vi "CalculateTrajectory2.vi"(9 "ChangingDistance":dbl, 10 "Inputs":T1, 11 "Lanes":T2) -> (2 "Trajectory":cluster{"X":dbl[], "Y":dbl[], "Theta":dbl[]})   [LabVIEW 2013]
uses:
  <vilib>/imath/engines/lvmath2/RunTimeEngine/ErrorHandling/NIMS_Finalize Error.vi
  <vilib>/imath/engines/lvmath2/RunTimeEngine/Managers/WorkSpace/UID Generator.vi
  <vilib>/imath/engines/lvmath2/RunTimeEngine/IndexRead/NIMS M($,S).vi
  <instcachedir>/0/NIMS M($,S)_3E5749BBB62E49528D4765A77F1F6D98.lvgen/NIMS M($,S)_3E5749BBB62E49528D4765A77F1F6D98_000.vi
  <vilib>/imathl/engines/lvmath/Functions/Error Handling/Create Error.vi
  <vilib>/imath/engines/lvmath2/RunTimeEngine/CommandStatement/NIMS_CommandStatement_MaskErr.vi
  <vilib>/imath/engines/lvmath2/RunTimeEngine/Managers/SymbolTable/Clear UID.vi
  <vilib>/imath/engines/lvmath2/RunTimeEngine/NodeEndStatement/NIMS_NodeEndStatement_Output.vi
  <instcachedir>/0/NIMS_NodeEndStatement_Output_53EC0D466D134D7ABD903AC30B43404B.lvgen/NIMS_NodeEndStatement_Output_53EC0D466D134D7ABD903AC30B43404B_005.vi
  <instcachedir>/0/NIMS_NodeEndStatement_Output_53EC0D466D134D7ABD903AC30B43404B.lvgen/NIMS_NodeEndStatement_Output_53EC0D466D134D7ABD903AC30B43404B_000.vi
  <vilib>/imath/engines/lvmath2/RunTimeEngine/IndexRead/NIMS V(S).vi
  <instcachedir>/0/NIMS V(S)_0488751826AF41519A22953C041130DC.lvgen/NIMS V(S)_0488751826AF41519A22953C041130DC_000.vi
  <vilib>/imath/engines/lvmath2/RunTimeEngine/ArithmeticOperatorToken/NIMS_ArithmeticOperator_plus.vi
  <instcachedir>/0/NIMS_ArithmeticOperator_plus_8A46DAFC24D445C9B2C97B626139369E.lvgen/NIMS_ArithmeticOperator_plus_8A46DAFC24D445C9B2C97B626139369E_004.vi
  <vilib>/imath/engines/lvmath2/RunTimeEngine/ErrorHandling/NIMS_Create Error From Enums.vi
  <vilib>/imath/engines/lvmath2/RunTimeEngine/BuiltInFunctions/min/1 input/NIMS_min(CV).vi
  <instcachedir>/0/NIMS_min(CV)_46E60952406B4159AB512BDF500C959F.lvgen/NIMS_min(CV)_46E60952406B4159AB512BDF500C959F_000.vi
  <vilib>/imath/engines/lvmath2/RunTimeEngine/CommandStatement/MC_CommandStatement_break.vi
  <vilib>/imath/engines/lvmath2/RunTimeEngine/BuiltInFunctions/length/NIMS_length(GV).vi
  <instcachedir>/0/NIMS_length(GV)_08A3D13377FD4E4B96F5795FBF3698FA.lvgen/NIMS_length(GV)_08A3D13377FD4E4B96F5795FBF3698FA_000.vi
  <vilib>/imath/engines/lvmath2/RunTimeEngine/IndexRead/NIMS V(R2).vi
  <instcachedir>/0/NIMS V(R2)_C76619605A0E4E9F8B2FA9389712AC47.lvgen/NIMS V(R2)_C76619605A0E4E9F8B2FA9389712AC47_000.vi
  <vilib>/imath/engines/lvmath2/RunTimeEngine/RunTimeType/NIMS_RunTimeType_From StrictType (excl LVString).vi
  <instcachedir>/0/NIMS_RunTimeType_From StrictType (excl LVString)_4DEE718D6EB74582AA20236969C084FC.lvgen/NIMS_RunTimeType_From StrictType (excl LVString)_4DEE718D6EB74582AA20236969C084FC_000.vi
  <vilib>/imath/engines/lvmath2/RunTimeEngine/LocalVariableDefStatement/MC_LocalVariableDefStatement_Display.vi
  <vilib>/imath/engines/lvmath2/RunTimeEngine/RangeToken/NIMS_Range.vi
  <instcachedir>/0/NIMS_Range_7481B155BEE341ECA0F59DDB444E2C09.lvgen/NIMS_Range_7481B155BEE341ECA0F59DDB444E2C09_000.vi
  <vilib>/imath/engines/lvmath2/RunTimeEngine/ArithmeticOperatorToken/NIMS_ArithmeticOperator_times.vi
  <instcachedir>/0/NIMS_ArithmeticOperator_times_F6527734CE75451889337B8CE94765C6.lvgen/NIMS_ArithmeticOperator_times_F6527734CE75451889337B8CE94765C6_002.vi
  <instcachedir>/0/NIMS_ArithmeticOperator_plus_8A46DAFC24D445C9B2C97B626139369E.lvgen/NIMS_ArithmeticOperator_plus_8A46DAFC24D445C9B2C97B626139369E_001.vi
  <vilib>/imath/engines/lvmath2/RunTimeEngine/BuiltInFunctions/difference/NIMS_difference(GV,I32).vi
  <instcachedir>/0/NIMS_difference(GV,I32)_DC7351DCBCF840A8AE147F50EC2CE86E.lvgen/NIMS_difference(GV,I32)_DC7351DCBCF840A8AE147F50EC2CE86E_001.vi
  <vilib>/imath/engines/lvmath2/RunTimeEngine/BuiltInFunctions/atan2/NIMS_atan2(A,A).vi
  <instcachedir>/0/NIMS_atan2(A,A)_2936FD7F864E46C682B467FE18724EF9.lvgen/NIMS_atan2(A,A)_2936FD7F864E46C682B467FE18724EF9_005.vi
  <vilib>/imath/engines/lvmath2/RunTimeEngine/Managers/SymbolTable/NIMS_WorkSpace.lvlib
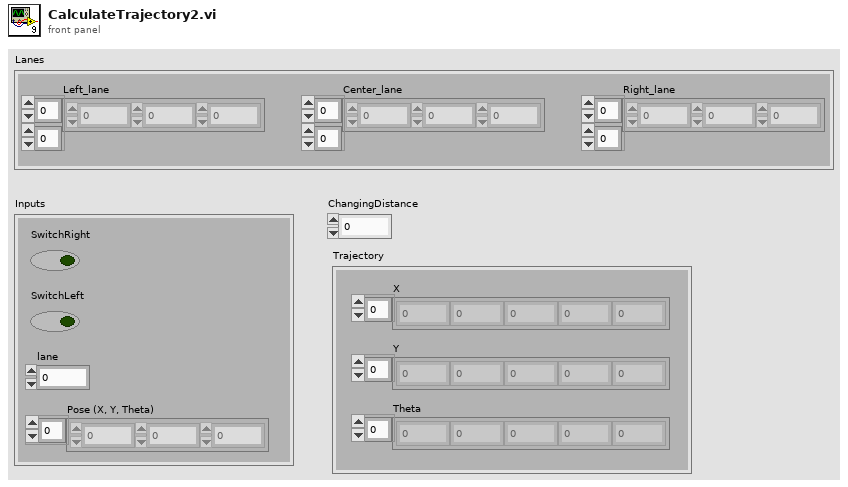
[diagram p1: front panel]
types:
  T1 = cluster{"Pose (X, Y, Theta)":dbl[], "lane":dbl, "SwitchRight":bool, "SwitchLeft":bool}
  T2 = cluster{"Right_lane":dbl[][], "Center_lane":dbl[][], "Left_lane":dbl[][]}
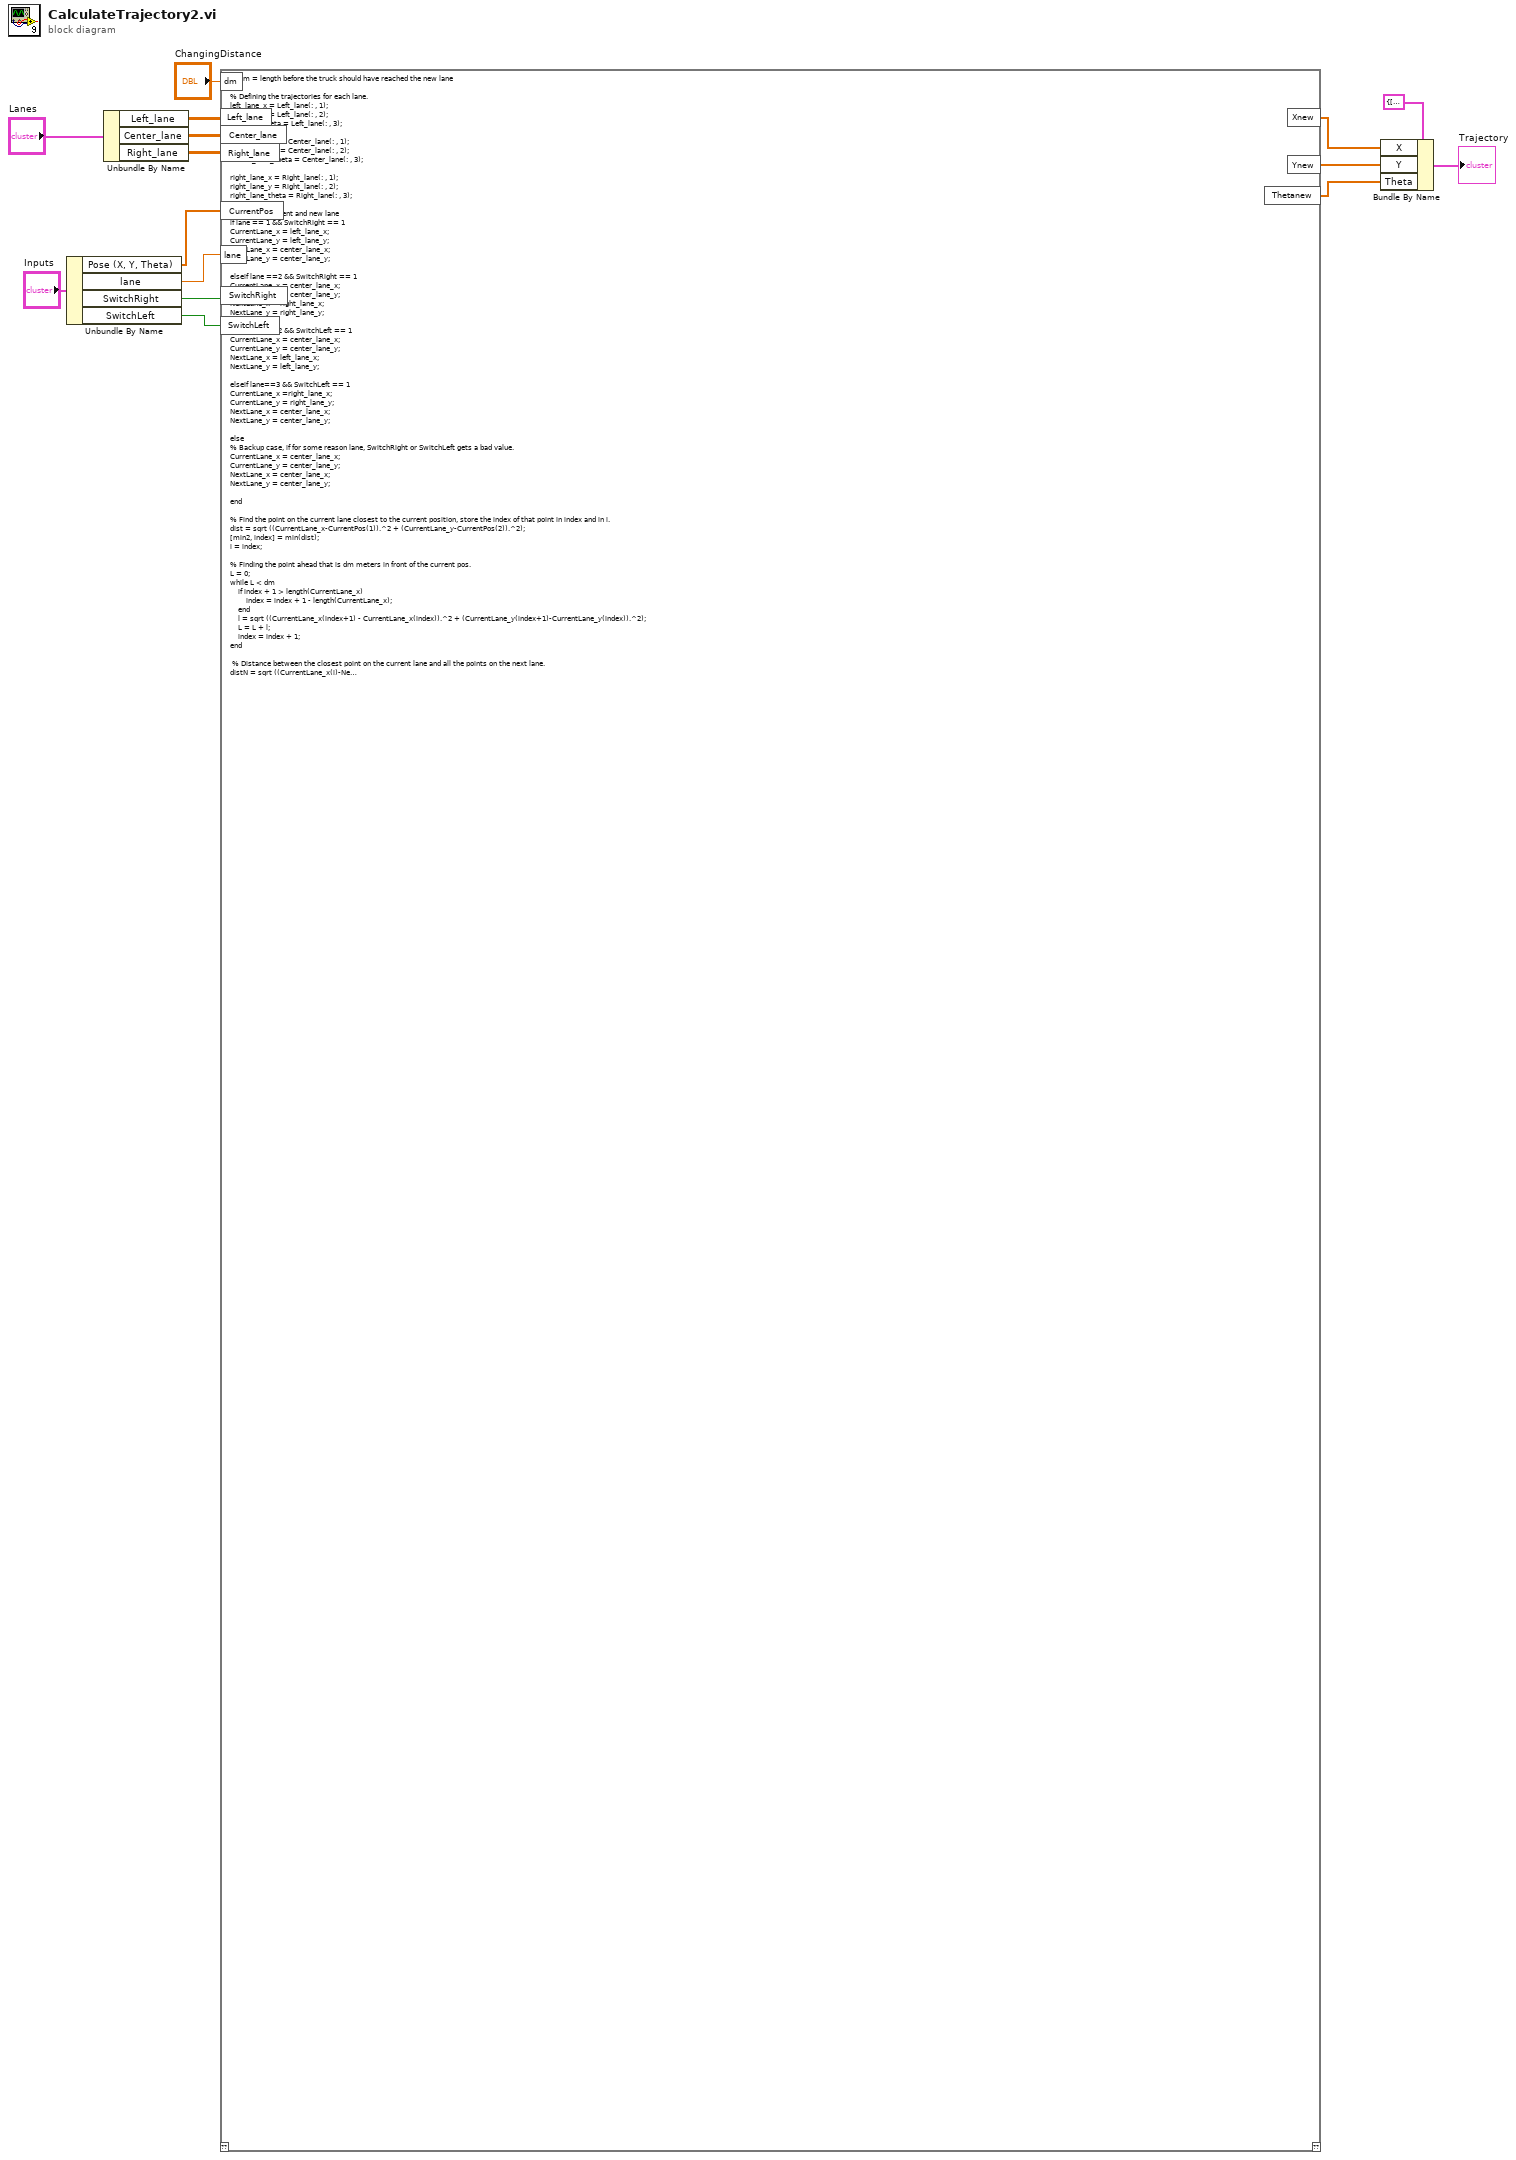
[diagram p0: block diagram]
diagram:
  n1 = Unbundle By Name("Inputs") -> ("Pose (X, Y, Theta)"=w11:dbl[], "lane"=w10:dbl, "SwitchRight"=w9:bool, "SwitchLeft"=w8:bool)
  n2 = Unbundle By Name("Lanes") -> ("Left_lane"=w15:dbl[][], "Center_lane"=w14:dbl[][], "Right_lane"=w13:dbl[][])
  n3 = mathscript code="% dm = length before the truck should have reached the new lane\n\n% Defining the trajectories for each lane.\nleft_lane_x = Left_lane(: , 1);\nleft_lane_y = Left_lane(: , 2);\nleft_lane_theta = Left_lane(: , 3);\n\ncenter_lane_x = Center_lane(: , 1);\ncenter_lane_y = Center_lane(: , 2);\ncenter_lane_theta = Center_lane(: , 3);\n\nright_lane_x = Right_lane(: , 1);\nright_lane_y = Right_lane(: , 2);\nright_lane_theta = Right_lane(: , 3);\n\n% Defining current and new lane\nif lane == 1 && SwitchRight == 1\nCurrentLane_x = left_lane_x;\nCurrentLane_y = left_lane_y;\nNextLane_x = center_lane_x;\nNextLane_y = center_lane_y;\n\nelseif lane ==2 && SwitchRight == 1\nCurrentLane_x = center_lane_x;\nCurrentLane_y = center_lane_y;\nNextLane_x = right_lane_x;\nNextLane_y = right_lane_y;\n\nelseif lane ==2 && SwitchLeft == 1\nCurrentLane_x = center_lane_x;\nCurrentLane_y = center_lane_y;\nNextLane_x = left_lane_x;\nNextLane_y = left_lane_y;\n\nelseif lane==3 && SwitchLeft == 1\nCurrentLane_x =right_lane_x;\nCurrentLane_y = right_lane_y;\nNextLane_x = center_lane_x;\nNextLane_y = center_lane_y;\n\nelse\n% Backup case, if for some reason lane, SwitchRight or SwitchLeft gets a bad value. \nCurrentLane_x = center_lane_x;\nCurrentLane_y = center_lane_y;\nNextLane_x = center_lane_x;\nNextLane_y = center_lane_y;\n\nend\n\n% Find the point on the current lane closest to the current position, store the index of that point in index and in i.\ndist = sqrt ((CurrentLane_x-CurrentPos(1)).^2 + (CurrentLane_y-CurrentPos(2)).^2);\n[min2, index] = min(dist);\ni = index;\n\n% Finding the point ahead that is dm meters in front of the current pos.\nL = 0;\nwhile L < dm\n    if index + 1 > length(CurrentLane_x)\n        index = index + 1 - length(CurrentLane_x);\n    end\n    l = sqrt ((CurrentLane_x(index+1) - CurrentLane_x(index)).^2 + (CurrentLane_y(index+1)-CurrentLane_y(index)).^2);\n    L = L + l;\n    index = index + 1;\nend\n\n % Distance between the closest point on the current lane and all the points on the next lane.\ndistN = sqrt ((CurrentLane_x(i)-NextLane_x).^2 + (CurrentLane_y(i)-NextLane_y).^2);\n% Distance between the ahead point on the current lane and all the points on the next lane.\ndistD = sqrt ((CurrentLane_x(index)-NextLane_x).^2 + (CurrentLane_y(index)-NextLane_y).^2);\n\n% IndexN is the index of the point on the next lane that is closest to the current pos.\n[minN, indexN] = min(distN); \n% IndexD is the index of the point on th next lane that is closest to the ahead point.\n[minD, indexD] = min(distD); \n\n% Create an array of the points on the current and the new lane that will be used for calculating the trajectory between them.\nif index < i\n    XnewC = [CurrentLane_x(i:length(CurrentLane_x))] \n    XnewC = [XnewC; CurrentLane_x(1:index)];\n    YnewC = [CurrentLane_y(i:length(CurrentLane_y))] \n    YnewC = [YnewC; CurrentLane_y(1:index)];\n else\n    XnewC = CurrentLane_x(i:index);\n    YnewC = CurrentLane_y(i:index);\nend\n\nif indexN > indexD\n    XnewN = [NextLane_x(indexN:length(NextLane_x)); NextLane_x(1:indexD)];\n    YnewN = [NextLane_y(indexN:length(NextLane_y)); NextLane_y(1:indexD)];\nelse\n     XnewN = NextLane_x(indexN:indexD);\n    YnewN = NextLane_y(indexN:indexD);\nend  \n\n% If the arrays have different dimensions, we need to add elements to the smaller one until they have the same length.\nd = length(XnewC)-length(XnewN);\nm = 0;\ni1 = 2;\nwhile m~=d\nsn = sign(d);\nm = m + sn*1;\n\nif sn < 0\n    b = XnewC(1);\n    c = YnewC(1);\n    XnewC = [XnewC(1); b; XnewC(2:end)];\n    YnewC = [YnewC(1); c; YnewC(2:end)];  \nelseif sn > 0\n    b = XnewN(1);\n    c = YnewN(1);\n    XnewN = [XnewN(1); b; XnewN(2:end)];\n    YnewN = [YnewN(1); c; YnewN(2:end)];\nend\nend\n\n% Use the weighted mean value to weight the new trajectory\n% weight = [1:(-1/(length(XnewC)-1)):0]';\n% weight_inverse = [0:(1/(length(XnewC)-1)):1]';\n\n% Use atan to weight the new trajectory\nsteg_inverse = [-1.5:(3/(length(XnewC)-1)):1.5];\nweight_inverse = [atan(steg_inverse)./(2*atan(1.5))+1/2]';\nsteg = [1.5:-(3/(length(XnewC)-1)):-1.5];\nweight = [atan(steg)./(2*atan(1.5))+1/2]';\n\n% Create the new trajectory between the lanes\nXnew =  (XnewC .* weight + XnewN .* weight_inverse);\nYnew = (YnewC .* weight + YnewN .* weight_inverse);\n\nThetanew = atan2(diff(Ynew), diff(Xnew));\nThetanew = [Thetanew' Thetanew(end)];"("Left_lane"=w15, "Center_lane"=w14, "Right_lane"=w13, "CurrentPos"=w11, "lane"=w10, "SwitchRight"=w9, "SwitchLeft"=w8, "dm"="ChangingDistance") -> ("Xnew"=w3:cdb[], "Ynew"=w2:cdb[], "Thetanew"=w1:dbl[])  [unwired: 1 in, 1 out]
  n4 = Bundle By Name(cluster=cluster{"X":dbl[], "Y":dbl[], "Theta":dbl[]} {"X"=[], "Y"=[], "Theta"=[]} ("Cluster"), "X"=w3, "Y"=w2, "Theta"=w1) -> (→"Trajectory":cluster{"X":dbl[], "Y":dbl[], "Theta":dbl[]})
